vi "Add Hardware.vi"(8 "error in (no error)":errorcluster, 10 "Mag Lab Hardware.lvclass":refnum<class "Mag Lab Hardware.lvclass">, 11 "Mag Lab Measure Controller in":refnum<class "Mag Lab Measure Controller.lvclass">) -> (0 "error out":errorcluster, 3 "Mag Lab Measure Controller out":refnum<class "Mag Lab Measure Controller.lvclass">)   [LabVIEW 2015, in "Mag Lab Measure Controller.lvclass"]
uses:
  Mag Lab Measure Controller.lvclass
  Hardware/Mag Lab Hardware.lvclass
  <vilib>/ActorFramework/Actor/Actor.lvclass/Actor.ctl
  <vilib>/ActorFramework/Message Enqueuer/Message Enqueuer.lvclass/Message Enqueuer.ctl
  Mag Lab Measure Controller.lvclass/Mag Lab Measure Controller.ctl
  Mag Lab Root/Mag Lab Root.lvclass/Mag Lab Root.ctl
  Mag Lab Measure Controller Messages/Log Status Update Msg/Log Status Update Msg.lvclass/Log Status Update Msg.ctl
  <vilib>/ActorFramework/Message Enqueuer/Init from Existing Queue.vi
  <vilib>/ActorFramework/Message Enqueuer/Enqueue.vi
  <vilib>/ActorFramework/Message Priority Queue/Priority Enqueue.vi
  <vilib>/ActorFramework/Message Enqueuer/Message Enqueuer.lvclass
  Mag Lab Measure Controller Messages/Log Status Update Msg/Log Status Update Msg.lvclass
  <vilib>/ActorFramework/Actor/Actor.lvclass
  Mag Lab Measure Base/Mag Lab Measure Base.lvclass
  Mag Lab Root/Mag Lab Root.lvclass
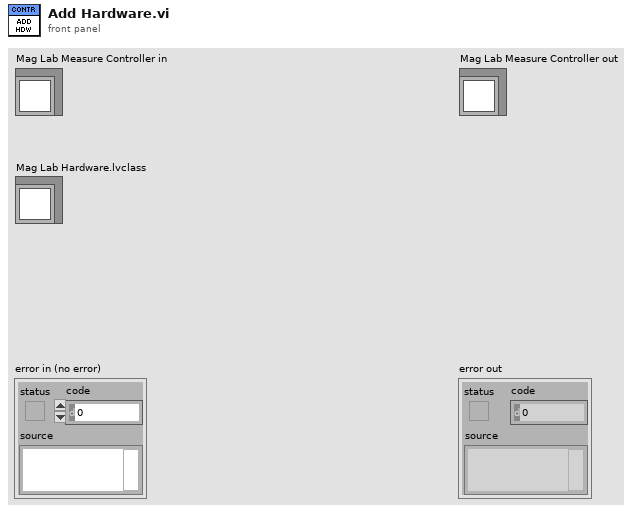
[diagram p1: front panel]
types:
  T1 = cluster{"Hardware Queue":refnum<class "Message Enqueuer.lvclass">, "Mag Lab Hardware.lvclass":refnum<class "Mag Lab Hardware.lvclass">}[]
  T2 = cluster{"Caller-To-Actor Enqueuer":refnum<class "Message Enqueuer.lvclass">, "Mag Lab Root out":refnum<class "Mag Lab Hardware.lvclass">}
  T3 = cluster{"Caller-To-Actor Enqueuer":refnum<class "Message Enqueuer.lvclass">, "Mag Lab Root out":refnum<class "Mag Lab Hardware.lvclass">}[]
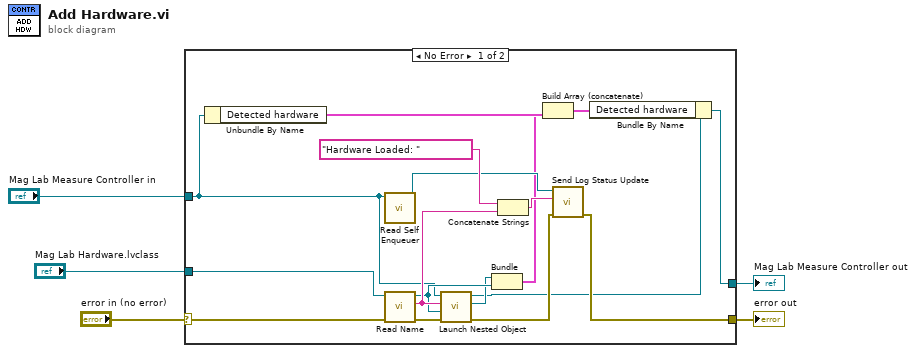
[diagram p0: block diagram]
diagram:
  n1 = case shown="No Error" "error in (no error)" {
    selector: "error in (no error)" -> [w14 w24]
    tunnel: [w19 w24] -> w4
    tunnel: [w7 w23] -> w2
    tunnel: "Mag Lab Measure Controller in" -> [w8 w23]
    tunnel: "Mag Lab Hardware.lvclass" -> [w15 _]
    frame No Error {
      n2 = Unbundle By Name(w8) -> ("Detected hardware"=w13:T1)
      n3 = call <vilib>:"Read Self Enqueuer.vi"("Actor"=w8) -> ("Self Enqueuer"=w20:refnum<class "Message Enqueuer.lvclass">)  [unwired: 10 in]
      n4 = call "Read Name.vi"("error in (no error)"=w14, "Mag Lab Root in"=w15) -> ("error out"=w16:errorcluster, "Name"=w18:string, "Mag Lab Root out"=w12:refnum<class "Mag Lab Hardware.lvclass">)  [unwired: 7 in]
      n5 = call "Launch Nested Object.vi"("error in (no error)"=w16, "Object"=w12, "name"=w18, "Mag Lab Measure Base in"=w8) -> ("error out"=w17:errorcluster, "Caller-To-Actor Enqueuer"=w11:refnum<class "Message Enqueuer.lvclass">, "Mag Lab Measure Base out"=w9:refnum<class "Mag Lab Measure Controller.lvclass">)  [unwired: 5 in]
      n6 = Bundle("Caller-To-Actor Enqueuer"=w11, "Mag Lab Root out"=w12) -> (w10:T2)  [unwired: 1 in]
      n7 = Concatenate Strings("Hardware Loaded: " ("string"), w18) -> (w21:string)
      n8 = Build Array (concatenate)(w13, w10) -> (w6:T3)
      n9 = call "Send Log Status Update.vi"("error in (no error)"=w17, "Status"=w21, "Message Enqueuer"=w20) -> ("error out"=w19:errorcluster)  [unwired: 7 in, 1 out]
      n10 = Bundle By Name(cluster=w9, "Detected hardware"=w6) -> (w7:refnum<class "Mag Lab Measure Controller.lvclass">)
    }
    frame Error {
    }
  }
  "error out" <- w4
  "Mag Lab Measure Controller out" <- w2
